vi "CleanUp.vi"(8 "error in (no error)":errorcluster, 11 "AjustesPrevios in":refnum<class "AjustesPrevios.lvclass">) -> (0 "error out":errorcluster, 3 "AjustesPrevios out":refnum<class "AjustesPrevios.lvclass">)   [LabVIEW 2019, in "AjustesPrevios.lvclass"]
uses:
  AjustesPrevios.lvclass
  AjustesPrevios.lvclass/AjustesPrevios.ctl
  Base de Datos/Base de Datos.lvclass
panel:
  out "Tabla":string[][](array[string])
  out "Voltaje enviado a CAM":dbl
  out "Humedad Relativa Aire [%]":dbl
  out "Presión Medida Pistófono  [hPa]":dbl
  out "Temperatura interna Pistófono[ºC]":dbl
  out "Nivel Emitido Pistófono [dB]":dbl
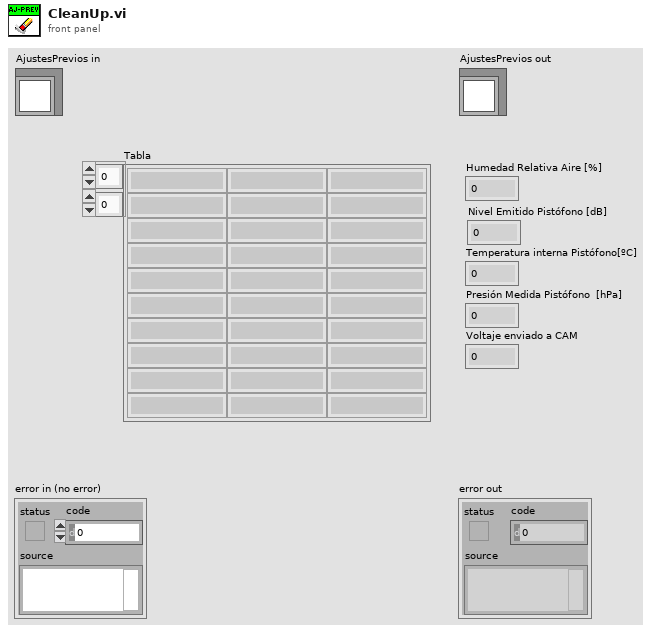
[diagram p1: front panel]
types:
  T1 = cluster{"igualacion_de_patrones":cluster{"Nivel Emitido Pistófono [dB]":dbl, "Temperatura interna Pistófono[ºC]":dbl, "Presión Medida Pistófono  [hPa]":dbl, "Humedad Relativa Aire [%]":dbl, "Factor de corrección de sensibilidad Nexus":dbl}, "Tabla Referencia Acústica Generador Externo":string[][], "Voltaje enviado a CAM":dbl, "usuario_registra":i32, "id_pon_frecuencia":i32}
  T2 = cluster{"Nivel Emitido Pistófono [dB]":dbl, "Temperatura interna Pistófono[ºC]":dbl, "Presión Medida Pistófono  [hPa]":dbl, "Humedad Relativa Aire [%]":dbl, "FactorCorreccionSensNexus":dbl}
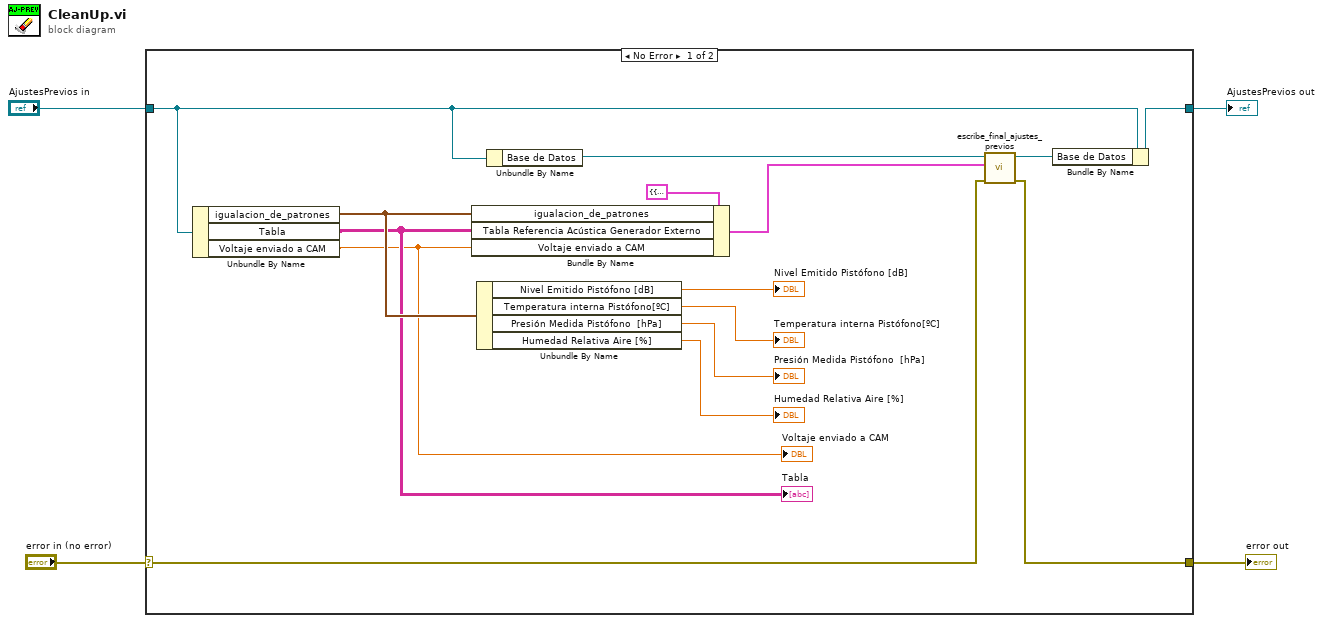
[diagram p0: block diagram]
diagram:
  n1 = case shown="No Error" "error in (no error)" {
    selector: "error in (no error)" -> [w5 w20]
    tunnel: "AjustesPrevios in" -> [w15 w21]
    tunnel: [w13 w21] -> w3
    tunnel: [w6 w20] -> w2
    frame No Error {
      n2 = Unbundle By Name(w15) -> ("igualacion_de_patrones"=w10:T2, "Tabla"=w8:string[][], "Voltaje enviado a CAM"=w7:dbl)
      "Voltaje enviado a CAM" <- w7
      "Tabla" <- w8
      n3 = Bundle By Name(cluster=T1 {"igualacion_de_patrones"={"Nivel Emitido Pistófono [dB]"=0.0, "Temperatura interna Pistófono[ºC]"=0.0, "Presión Medida Pistófono  [hPa]"=0.0, "Humedad Relativa Aire [%]"=0.0, "Factor de corrección de sensibilidad Nexus"=0.0}, "Tabla Referencia Acústica Generador Externo"=[], "Voltaje enviado a CAM"=0.0, "usuario_registra"=1, "id_pon_frecuencia"=0} ("Datos a Escribir"), "igualacion_de_patrones"=w10, "Tabla Referencia Acústica Generador Externo"=w8, "Voltaje enviado a CAM"=w7) -> (w9:T1)
      n4 = Unbundle By Name(w10) -> ("Nivel Emitido Pistófono [dB]"=→"Nivel Emitido Pistófono [dB]":dbl, "Temperatura interna Pistófono[ºC]"=→"Temperatura interna Pistófono[ºC]":dbl, "Presión Medida Pistófono  [hPa]"=→"Presión Medida Pistófono  [hPa]":dbl, "Humedad Relativa Aire [%]"=→"Humedad Relativa Aire [%]":dbl)
      n5 = Unbundle By Name(w15) -> ("Base de Datos"=w14:refnum<class "Base de Datos.lvclass">)
      n6 = call "escribe_final_ajustes_previos.vi"("error in (no error)"=w5, "Datos a Escribir"=w9, "DB in"=w14) -> ("error out"=w6:errorcluster, "DB out"=w12:refnum<class "Base de Datos.lvclass">)  [unwired: 7 in]
      n7 = Bundle By Name(cluster=w15, "Base de Datos"=w12) -> (w13:refnum<class "AjustesPrevios.lvclass">)
    }
    frame Error {
    }
  }
  "error out" <- w2
  "AjustesPrevios out" <- w3
